vi "saveDataNodeBegin.vi"(8 "error in (no error)":errorcluster, 9 "indent":i32, 10 "XML Refnum in":refnum<file>, 11 "DMA_Read in":refnum<class "DMA_Read.lvclass">) -> (0 "error out":errorcluster, 2 "XML Refnum out":refnum<file>, 3 "DMA_Read out":refnum<class "DMA_Read.lvclass">)   [LabVIEW 2013, in "DMA_Read.lvclass"]
doc: "Begins the process of saving a xceData Node to an XML formatted file."
uses:
  DMA_Read.lvclass
  xCE/xceNode/xceNode.lvclass
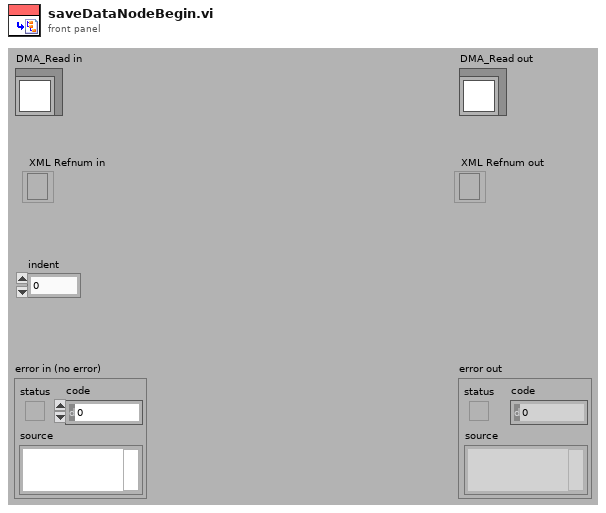
[diagram p1: front panel]
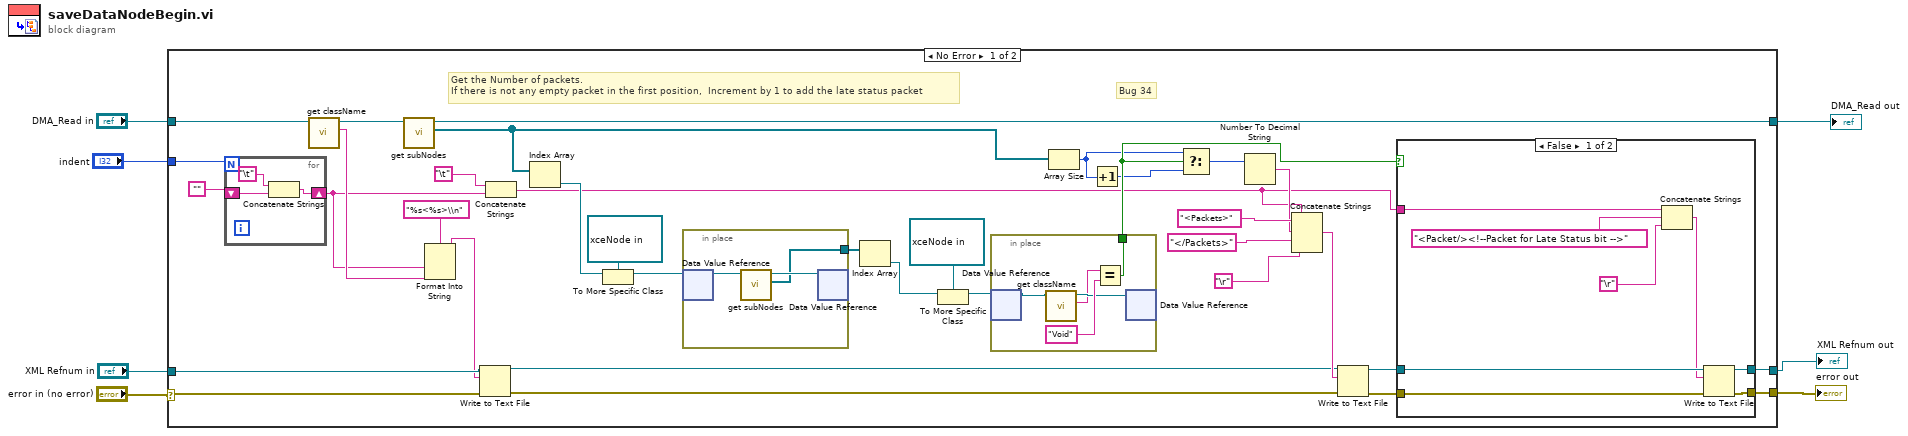
[diagram p0: block diagram]
diagram:
  n1 = case shown="No Error" "error in (no error)" {
    selector: "error in (no error)" -> [w30 w67]
    tunnel: "XML Refnum in" -> [w32 w66]
    tunnel: [w26 w67] -> w5
    tunnel: [w25 w66] -> w4
    tunnel: "DMA_Read in" -> [w36 w65]
    tunnel: [w13 w65] -> w2
    tunnel: "indent" -> [w42 _]
    frame No Error {
      # "Bug 34"
      # "Get the Number of packets.\nIf there is not any empty packet in the first position,  Increment by 1 to add the late status packet"
      n2 = for {
        N: w42 -> [_]
        shift-right: [w64] -> w34
        shift-left: "" -> [w63]
        n3 = Concatenate Strings("\t", w63) -> (w64:string)
      }
      n4 = call "get className.vi"("xceNode in"=w36) -> ("Class name"=w35:string, "xceNode out"=w22:refnum<class "DMA_Read.lvclass">)  [unwired: 8 in, 1 out]
      n5 = call "get subNodes.vi"("xceNode in"=w22) -> ("subNodes[]*"=w14:refnum<data-value>[], "xceNode out"=w13:refnum<class "DMA_Read.lvclass">)  [unwired: 8 in, 1 out]
      n6 = Format Into String(format string="%s<%s>\\n", w34, w35) -> (resulting string=w31:string)  [unwired: 2 in, 1 out]
      n7 = Write to Text File(file (use dialog)=w32, text=w31, error in=w30) -> (refnum out=w29:refnum<file>, error out=w28:errorcluster)  [unwired: 1 in, 1 out]
      n8 = Concatenate Strings("\t", w34) -> (w8:string)
      n9 = Index Array(array=w14) -> (element=w20:refnum<data-value>)  [unwired: 1 in]
      n10 = To More Specific Class(target class=refnum<data-value> refnum ("data value reference"), reference=w20) -> (specific class reference=w19:refnum<data-value>)  [unwired: 1 in, 1 out]
      n11 = in-place {
        in-place-border: [w49] -> w18
        n12 = in-place-dvr #1(w19) -> (w51:refnum<class "xceNode.lvclass">)  [unwired: 1 out]
        n13 = call "get subNodes.vi"("xceNode in"=w51) -> ("subNodes[]*"=w49:refnum<data-value>[], "xceNode out"=w50:refnum<class "xceNode.lvclass">)  [unwired: 8 in, 1 out]
        n14 = in-place-dvr #1(w50) -> ()  [unwired: 2 out]
      }
      n15 = Index Array(array=w18) -> (element=w16:refnum<data-value>)  [unwired: 1 in]
      n16 = To More Specific Class(target class=refnum<data-value> refnum ("data value reference"), reference=w16) -> (specific class reference=w15:refnum<data-value>)  [unwired: 1 in, 1 out]
      n17 = in-place {
        in-place-border: [w47] -> w12
        n18 = in-place-dvr #2(w15) -> (w46:refnum<class "xceNode.lvclass">)  [unwired: 1 out]
        n19 = call "get className.vi"("xceNode in"=w46) -> ("Class name"=w44:string, "xceNode out"=w45:refnum<class "xceNode.lvclass">)  [unwired: 8 in, 1 out]
        n20 = Equal?(x=w44, y="Void") -> (x = y?=w47:bool)
        n21 = in-place-dvr #2(w45) -> ()  [unwired: 2 out]
      }
      n22 = Array Size(array=w14) -> (size(s)=w9:i32)
      n23 = Increment(x=w9) -> (x+1=w11:i32)
      n24 = Select(t=w9, s=w12, f=w11) -> (s? t:f=w10:i32)
      n25 = Number To Decimal String(number=w10) -> (decimal integer string=w39:string)  [unwired: 1 in]
      n26 = Concatenate Strings(w8, "<Packets>" ("string"), w39, "</Packets>" ("string"), "\r") -> (w38:string)
      n27 = Write to Text File(file (use dialog)=w29, text=w38, error in=w28) -> (refnum out=w23:refnum<file>, error out=w24:errorcluster)  [unwired: 1 in, 1 out]
      n28 = case shown="False" w12 {
        tunnel: [w59 w60] -> w26
        tunnel: [w58 w61] -> w25
        tunnel: w24 -> [w57 w60]
        tunnel: w23 -> [w56 w61]
        tunnel: w8 -> [w54 _]
        frame False {
          n29 = Concatenate Strings(w54, "<Packet/><!--Packet for Late Status bit -->" ("string"), "\r") -> (w52:string)
          n30 = Write to Text File(file (use dialog)=w56, text=w52, error in=w57) -> (refnum out=w58:refnum<file>, error out=w59:errorcluster)  [unwired: 1 in, 1 out]
        }
        frame True {
        }
      }
    }
    frame Error {
    }
  }
  "error out" <- w5
  "DMA_Read out" <- w2
  "XML Refnum out" <- w4
